vi "OP300ZP_TIMER.vi"() -> ()   [LabVIEW 2020]
panel:
  in  "TIMER":dbl
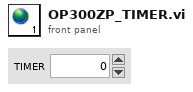
[diagram p1: front panel]
diagram:
